vi "Notify.vi"(8 "Error In":errorcluster, 10 "Message":string, 11 "reference in":refnum<class "Colleague.lvclass">) -> (0 "Error Out":errorcluster, 3 "reference out":refnum<class "Colleague.lvclass">)   [LabVIEW 2020, in "Colleague.lvclass"]
uses:
  Colleague.lvclass
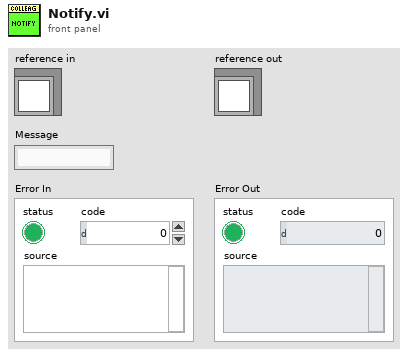
[diagram p1: front panel]
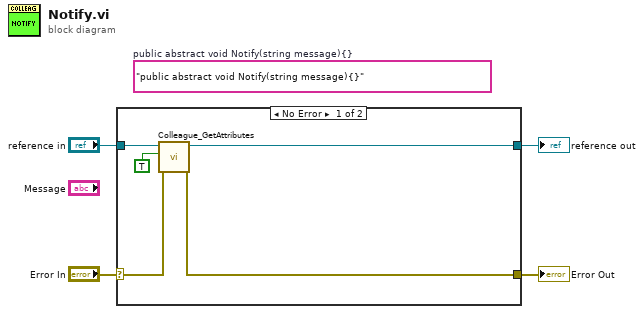
[diagram p0: block diagram]
diagram:
  (unwired) "public abstract void Notify(string message){}"  # public abstract void Notify(string message){}
  n1 = case shown="No Error" "Error In" {
    selector: "Error In" -> [w8 w11]
    tunnel: [w5 w11] -> w3
    tunnel: [w7 w10] -> w1
    tunnel: "reference in" -> [w9 w10]
    frame No Error {
      n2 = call "Colleague_GetAttributes.vi"("error in (no error)"=w8, "OnlyGetDvrReference(False)"=TRUE, "reference in"=w9) -> ("error out"=w5:errorcluster, "reference out"=w7:refnum<class "Colleague.lvclass">)  [unwired: 5 in, 2 out]
    }
    frame Error {
    }
  }
  "Error Out" <- w3
  "reference out" <- w1
